vi "generate student data.vi"(1 "number of class courses":i32, 2 "classes per student":i32, 3 "number of students":i32) -> (0 "Student data":i32[][](array[numeric]))   [LabVIEW 2009]
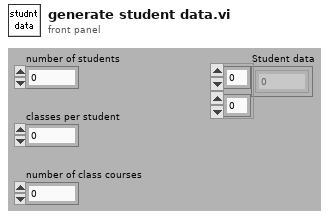
[diagram p1: front panel]
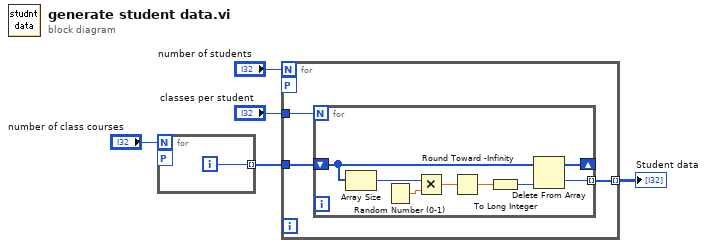
[diagram p0: block diagram]
diagram:
  n1 = for {
    N: "number of class courses" -> [_]
    tunnel: [w6] -> w1 mode=indexing
    workers-P: _ -> [_]
    i -> [w6]
  }
  n2 = for {
    N: "number of students" -> [_]
    tunnel: "classes per student" -> [w9]
    tunnel: w1 -> [w8]
    tunnel: [w7] -> w5 mode=indexing
    workers-P: _ -> [_]
    n3 = for {
      N: w9 -> [_]
      shift-right: [w15] -> _
      shift-left: w8 -> [w17]
      tunnel: [w16] -> w7 mode=indexing
      n4 = Array Size(array=w17) -> (size(s)=w14:i32)
      n5 = Random Number (0-1)() -> (number: 0 to 1=w13:dbl)
      n6 = Multiply(x=w14, y=w13) -> (x*y=w12:dbl)
      n7 = Round Toward -Infinity(1:w12) -> (0:w10:dbl)
      n8 = To Long Integer(number=w10) -> (32bit integer=w11:i32)
      n9 = Delete From Array(array=w17, index=w11) -> (deleted portion=w16:i32, array with subset deleted=w15:i32[])  [unwired: 1 in]
    }
  }
  "Student data" <- w5
